vi "Find Target.vi"(11 "Input":timestamp=timestamp(3614009430.8933406 s since 1904-01-01)) -> (3 "Is 2nd Tuesday of the Month?":bool)   [LabVIEW 2018, in "Tests.lvlib" / "Toolkit.lvlib" / "Integration.lvlib"]
uses:
  Integration.lvlib
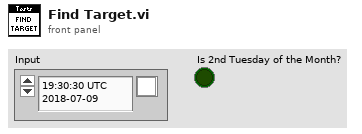
[diagram p1: front panel]
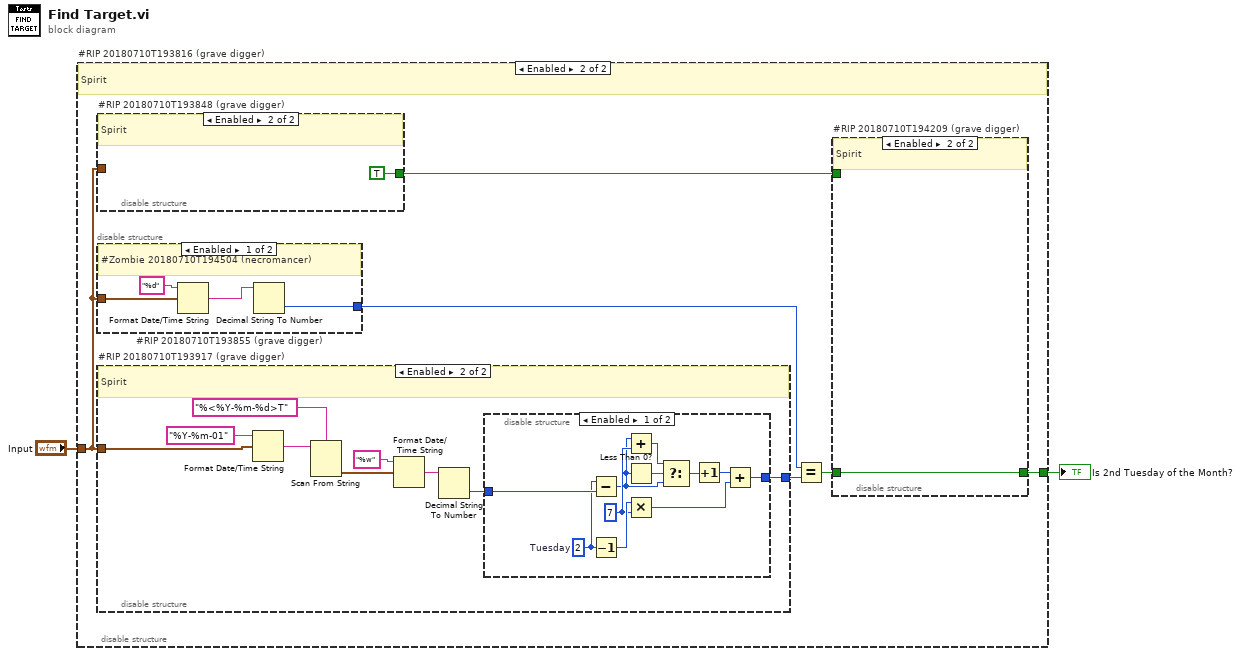
[diagram p0: block diagram]
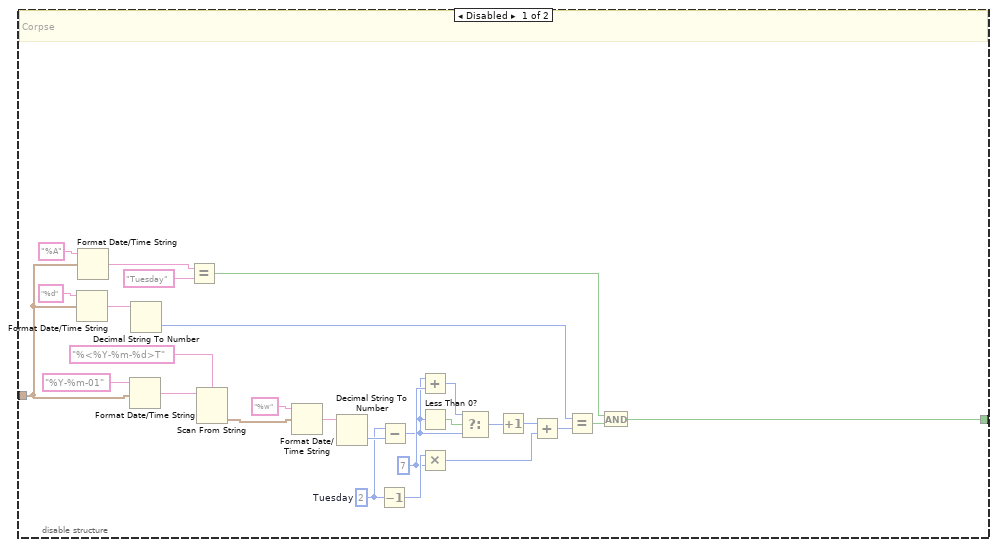
[diagram p2: hidden frame]
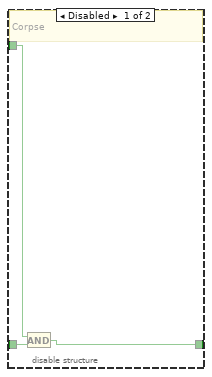
[diagram p3: hidden frame]
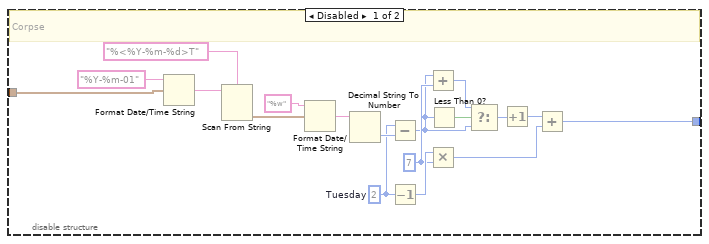
[diagram p4: hidden frame]
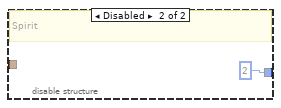
[diagram p6: hidden frame]
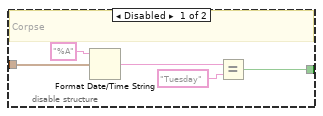
[diagram p7: hidden frame]
diagram:
  n1 = disable-structure "#RIP 20180710T193816 (grave digger)" shown="Enabled" {
    disable-tunnel: [w4 w31] -> w1
    disable-tunnel: "Input" -> [w3 w30]
    frame Disabled {
      w15 = 7
      w17 = 2  # Tuesday
      # "Corpse"
      n2 = Format Date/Time String(time format string (%c)="%d", seconds (now)=w3) -> (date/time string=w27:string)  [unwired: 1 in]
      n3 = Format Date/Time String(time format string (%c)="%A", seconds (now)=w3) -> (date/time string=w26:string)  [unwired: 1 in]
      n4 = Format Date/Time String(time format string (%c)="%Y-%m-01", seconds (now)=w3) -> (date/time string=w22:string)  [unwired: 1 in]
      n5 = Decimal String To Number(string=w27) -> (number=w6:i32)  [unwired: 2 in, 1 out]
      n6 = Equal?(x=w26, y="Tuesday") -> (x = y?=w8:bool)
      n7 = Scan From String(format string="%<%Y-%m-%d>T", input string=w22) -> (output 1=w21:timestamp)  [unwired: 3 in, 3 out]
      n8 = Format Date/Time String(time format string (%c)="%w", seconds (now)=w21) -> (date/time string=w19:string)  [unwired: 1 in]
      n9 = Decimal String To Number(string=w19) -> (number=w18:i32)  [unwired: 2 in, 1 out]
      n10 = Decrement(x=w17) -> (x-1=w16:i32)
      n11 = Subtract(x=w17, y=w18) -> (x-y=w12:i32)
      n12 = Add(x=w12, y=w15) -> (x+y=w13:i32)
      n13 = Less Than 0?(x=w12) -> (x < 0?=w14:bool)
      n14 = Multiply(x=w16, y=w15) -> (x*y=w9:i32)
      n15 = Select(t=w13, s=w14, f=w12) -> (s? t:f=w11:i32)
      n16 = Increment(x=w11) -> (x+1=w10:i32)
      n17 = Add(x=w10, y=w9) -> (x+y=w7:i32)
      n18 = Equal?(x=w6, y=w7) -> (x = y?=w5:bool)
      n19 = And(x=w8, y=w5) -> (x .and. y?=w4:bool)
    }
    frame Enabled {
      # "Spirit"
      n20 = disable-structure "#RIP 20180710T193848 (grave digger)" shown="Enabled" {
        disable-tunnel: [w85 TRUE] -> w35
        disable-tunnel: w30 -> [w84 _]
        frame Disabled {
          # "Corpse"
          n21 = Format Date/Time String(time format string (%c)="%A", seconds (now)=w84) -> (date/time string=w87:string)  [unwired: 1 in]
          n22 = Equal?(x=w87, y="Tuesday") -> (x = y?=w85:bool)
        }
        frame Enabled {
          # "Spirit"
        }
      }
      n23 = disable-structure "#RIP 20180710T193855 (grave digger)" shown="Enabled" {
        disable-tunnel: [w80 2] -> w33
        disable-tunnel: w30 -> [w79 _]
        frame Enabled {
          # "#Zombie 20180710T194504 (necromancer)"
          n24 = Format Date/Time String(time format string (%c)="%d", seconds (now)=w79) -> (date/time string=w81:string)  [unwired: 1 in]
          n25 = Decimal String To Number(string=w81) -> (number=w80:i32)  [unwired: 2 in, 1 out]
        }
        frame Disabled {
          # "Spirit"
        }
      }
      n26 = disable-structure "#RIP 20180710T193917 (grave digger)" shown="Enabled" {
        disable-tunnel: [w41 w59] -> w34
        disable-tunnel: w30 -> [w40 w58]
        frame Disabled {
          w48 = 7
          w50 = 2  # Tuesday
          # "Corpse"
          n27 = Format Date/Time String(time format string (%c)="%Y-%m-01", seconds (now)=w40) -> (date/time string=w55:string)  [unwired: 1 in]
          n28 = Scan From String(format string="%<%Y-%m-%d>T", input string=w55) -> (output 1=w54:timestamp)  [unwired: 3 in, 3 out]
          n29 = Format Date/Time String(time format string (%c)="%w", seconds (now)=w54) -> (date/time string=w52:string)  [unwired: 1 in]
          n30 = Decimal String To Number(string=w52) -> (number=w51:i32)  [unwired: 2 in, 1 out]
          n31 = Subtract(x=w50, y=w51) -> (x-y=w45:i32)
          n32 = Decrement(x=w50) -> (x-1=w49:i32)
          n33 = Add(x=w45, y=w48) -> (x+y=w46:i32)
          n34 = Multiply(x=w49, y=w48) -> (x*y=w42:i32)
          n35 = Less Than 0?(x=w45) -> (x < 0?=w47:bool)
          n36 = Select(t=w46, s=w47, f=w45) -> (s? t:f=w44:i32)
          n37 = Increment(x=w44) -> (x+1=w43:i32)
          n38 = Add(x=w43, y=w42) -> (x+y=w41:i32)
        }
        frame Enabled {
          # "Spirit"
          n39 = Format Date/Time String(time format string (%c)="%Y-%m-01", seconds (now)=w58) -> (date/time string=w64:string)  [unwired: 1 in]
          n40 = Scan From String(format string="%<%Y-%m-%d>T", input string=w64) -> (output 1=w63:timestamp)  [unwired: 3 in, 3 out]
          n41 = Format Date/Time String(time format string (%c)="%w", seconds (now)=w63) -> (date/time string=w61:string)  [unwired: 1 in]
          n42 = Decimal String To Number(string=w61) -> (number=w60:i32)  [unwired: 2 in, 1 out]
          n43 = disable-structure shown="Enabled" {
            disable-tunnel: w60 -> [w77 w78]
            disable-tunnel: [w67 w78] -> w59
            frame Enabled {
              w74 = 7
              w76 = 2  # Tuesday
              n44 = Subtract(x=w76, y=w77) -> (x-y=w71:i32)
              n45 = Decrement(x=w76) -> (x-1=w75:i32)
              n46 = Add(x=w71, y=w74) -> (x+y=w72:i32)
              n47 = Less Than 0?(x=w71) -> (x < 0?=w73:bool)
              n48 = Multiply(x=w75, y=w74) -> (x*y=w68:i32)
              n49 = Select(t=w72, s=w73, f=w71) -> (s? t:f=w70:i32)
              n50 = Increment(x=w70) -> (x+1=w69:i32)
              n51 = Add(x=w69, y=w68) -> (x+y=w67:i32)
            }
            frame Disabled {
            }
          }
        }
      }
      n52 = Equal?(x=w33, y=w34) -> (x = y?=w32:bool)
      n53 = disable-structure "#RIP 20180710T194209 (grave digger)" shown="Enabled" {
        disable-tunnel: w35 -> [w38 _]
        disable-tunnel: w32 -> [w37 w39]
        disable-tunnel: [w36 w39] -> w31
        frame Disabled {
          # "Corpse"
          n54 = And(x=w38, y=w37) -> (x .and. y?=w36:bool)
        }
        frame Enabled {
          # "Spirit"
        }
      }
    }
  }
  "Is 2nd Tuesday of the Month?" <- w1
